vi "test_cRIO daqmx Temp pure.vi"() -> ()   [LabVIEW 2023]
uses:
  Thermometer/Thermometer DAQmx Base CFG/Thermometer DAQmx Base CFG.lvclass
  D:/git/HAL/HAL GOOP4/Configuration/Configuration JSON/Configuration JSON Base/CFG JSON.lvclass
  Configuration/Configuration JSON/Configuration JSON Base/CFG JSON.lvclass
panel:
  out "Waveform Chart":dbl(graph)
  out "error out":errorcluster
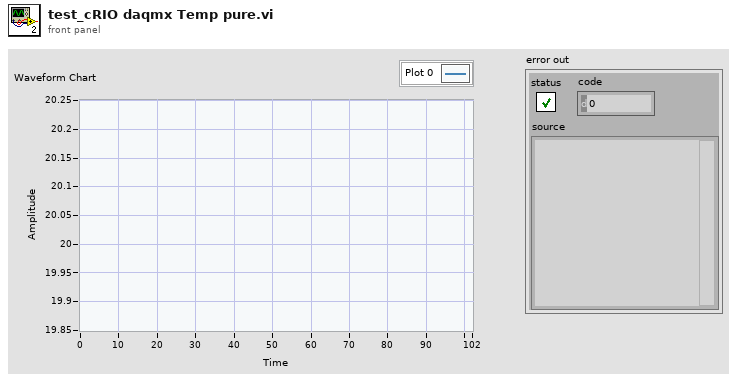
[diagram p1: front panel]
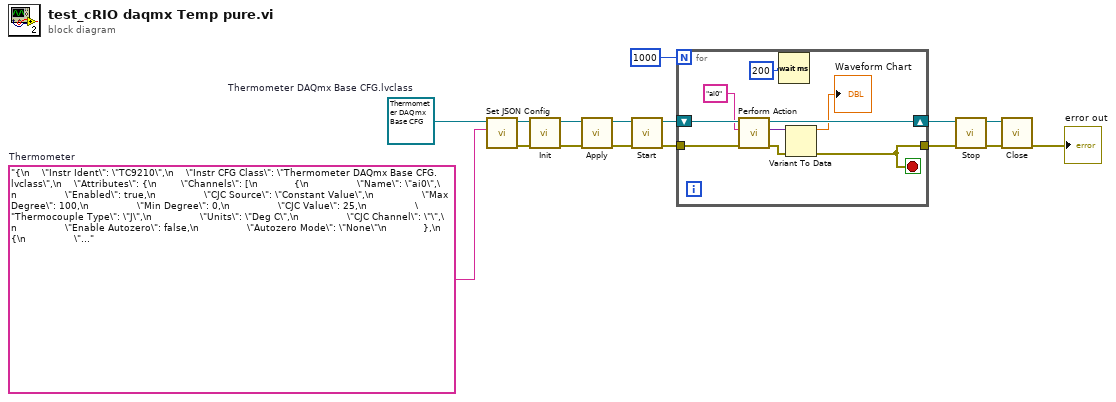
[diagram p0: block diagram]
diagram:
  w14 = "{\n    \"Instr Ident\": \"TC9210\",\n    \"Instr CFG Class\": \"Thermometer DAQmx Base CFG.lvclass\",\n    \"Attributes\": {\n        \"Channels\": [\n            {\n                \"Name\": \"ai0\",\n                \"Enabled\": true,\n                \"CJC Source\": \"Constant Value\",\n                \"Max Degree\": 100,\n                \"Min Degree\": 0,\n                \"CJC Value\": 25,\n                \"Thermocouple Type\": \"J\",\n                \"Units\": \"Deg C\",\n                \"CJC Channel\": \"\",\n                \"Enable Autozero\": false,\n                \"Autozero Mode\": \"None\"\n            },\n            {\n                \"Name\": \"ai1\",\n                \"Enabled\": false,\n                \"CJC Source\": \"Constant Value\",\n                \"Max Degree\": 100,\n                \"Min Degree\": 0,\n                \"CJC Value\": 25,\n                \"Thermocouple Type\": \"J\",\n                \"Units\": \"Deg C\",\n                \"CJC Channel\": \"\",\n                \"Enable Autozero\": false,\n                \"Autozero Mode\": \"None\"\n            },\n            {\n                \"Name\": \"ai2\",\n                \"Enabled\": false,\n                \"CJC Source\": \"Constant Value\",\n                \"Max Degree\": 100,\n                \"Min Degree\": 0,\n                \"CJC Value\": 25,\n                \"Thermocouple Type\": \"J\",\n                \"Units\": \"Deg C\",\n                \"CJC Channel\": \"\",\n                \"Enable Autozero\": false,\n                \"Autozero Mode\": \"None\"\n            },\n            {\n                \"Name\": \"ai3\",\n                \"Enabled\": false,\n                \"CJC Source\": \"Constant Value\",\n                \"Max Degree\": 100,\n                \"Min Degree\": 0,\n                \"CJC Value\": 25,\n                \"Thermocouple Type\": \"J\",\n                \"Units\": \"Deg C\",\n                \"CJC Channel\": \"\",\n                \"Enable Autozero\": false,\n                \"Autozero Mode\": \"None\"\n            }\n        ],\n        \"Timing\": {\n            \"Samples per Channel\": 1000,\n            \"Sample Mode\": \"Continuous Samples\",\n            \"Sample Rate\": 14,\n            \"Sample Clock Source\": \"OnboardClock\",\n            \"Active Edge\": \"Rising\"\n        },\n        \"Trigger\": {\n            \"Trigger Type\": \"No Trigger\"\n        },\n        \"Acquisition\": {\n            \"Relative To\": \"Current Read Position\",\n            \"Overwrite\": \"Do Not Overwrite Unread Samples\",\n            \"Samples per Fetch\": -1,\n            \"Timeout\": 1\n        }\n    }\n}"  # Thermometer
  w15 = refnum<class "Thermometer DAQmx Base CFG.lvclass"> refnum  # Thermometer DAQmx Base CFG.lvclass
  n1 = call "Set JSON Config.vi"("<JSON>Config>"=w14, "CFG Base in"=w15) -> ("error out"=w10:errorcluster, "CFG Base out"=w16:refnum<class "Thermometer DAQmx Base CFG.lvclass">)  [unwired: 8 in]
  n2 = call-dynamic "Init.vi"("error in (no error)"=w10, "DAQmx Base CFG in"=w16) -> ("error out"=w13:errorcluster, "DAQmx Base CFG out"=w11:refnum<class "Thermometer DAQmx Base CFG.lvclass">)  [unwired: 8 in]
  n3 = call-dynamic "Apply.vi"("error in (no error)"=w13, "DAQmx Base CFG in"=w11) -> ("error out"=w12:errorcluster, "DAQmx Base CFG out"=w9:refnum<class "Thermometer DAQmx Base CFG.lvclass">)  [unwired: 8 in]
  n4 = call-dynamic "Start.vi"("error in (no error)"=w12, "DAQmx Base CFG in"=w9) -> ("error out"=w8:errorcluster, "DAQmx Base CFG out"=w6:refnum<class "Thermometer DAQmx Base CFG.lvclass">)  [unwired: 8 in]
  n5 = for {
    N: 1000 -> [_]
    tunnel: w8 -> [w25]
    tunnel: [w20] -> w7
    shift-right: [w21] -> w3
    shift-left: w6 -> [w23]
    stop <- w20 stop-if-true
    n6 = call-dynamic "Perform Action.vi"("error in (no error)"=w25, "Input"="ai0", "Thermometer DAQmx Base CFG in"=w23) -> ("error out"=w24:errorcluster, "Output"=w19:variant, "Thermometer DAQmx Base CFG out"=w21:refnum<class "Thermometer DAQmx Base CFG.lvclass">)  [unwired: 6 in]
    n7 = Wait (ms)(milliseconds to wait=u32 200) -> ()  [unwired: 1 out]
    n8 = Variant To Data(error in=w24, Variant=w19) -> (data=→"Waveform Chart":dbl, error out=w20:errorcluster)  [unwired: 1 in]
  }
  n9 = call-dynamic "Stop.vi"("error in (no error)"=w7, "DAQmx Base CFG in"=w3) -> ("error out"=w4:errorcluster, "DAQmx Base CFG out"=w1:refnum<class "Thermometer DAQmx Base CFG.lvclass">)  [unwired: 8 in]
  n10 = call-dynamic "Close.vi"("error in (no error)"=w4, "Thermometer DAQmx Base CFG in"=w1) -> ("error out"=→"error out":errorcluster)  [unwired: 8 in, 1 out]
